vi "ZE_Recorder_AddHeaderToFile.vi"(4 "property values":string[](array[string]), 6 "property names":string[](array[string]), 7 "Header in":string, 8 "error in":errorcluster caption="error in (no error)", 9 "File Type":enum32{"CSV", "TDMS"}(ring), 10 "tdms refnum":refnum<k34>, 11 "csv refnum in":refnum<file>) -> (0 "error out":errorcluster)   [LabVIEW 2025, in "ZE_Recorder.lvlib"]
doc: "ZE_Recorder_AddHeaderToFile.vi\n----------------------------------------------\nThe VI adds a file header containing the measurement information to a CSV or TDMS file.\n\nInputs:\n---------------------\n- property values : 1DArrayOfString; \n- property names : 1DArrayOfString; \n- Header in : String; \n- error in (no error) : Cluster; \n- File Type : EnumU32; \n- tdms refnum : Refnum; \n- csv refnum in : Refnum; \n\nOutputs:\n---------------------\n- error out : Cluster; \n\n----------------------------------------------\n13.06.2016\nZühlke Engineering AG\nCH-8952 Schlieren\nwww.zuehlke.com"
uses:
  ZE_Recorder.lvlib
panel:
  # "Connector Pane"
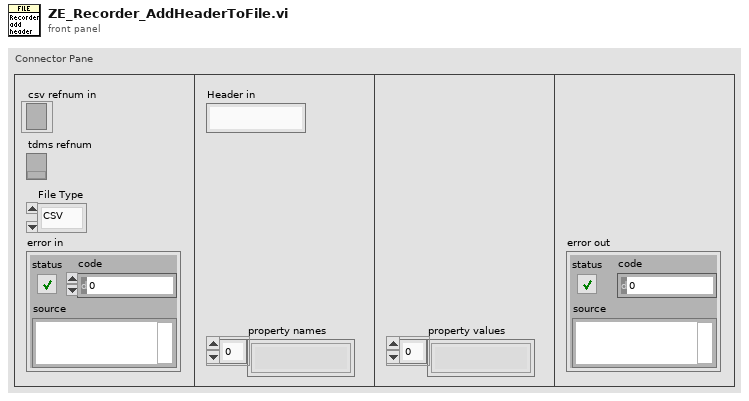
[diagram p1: front panel]
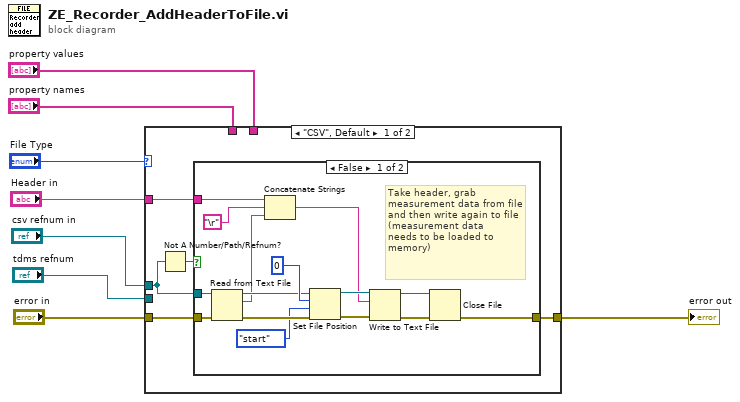
[diagram p0: block diagram]
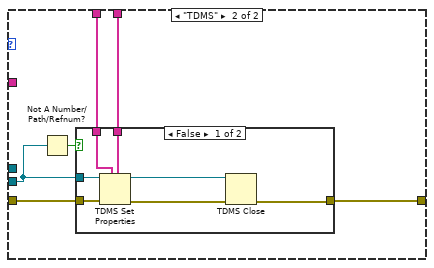
[diagram p3: hidden frame]
diagram:
  n1 = case shown="\"CSV\", Default" "File Type" {
    tunnel: "csv refnum in" -> [w10 _]
    tunnel: "error in" -> [w12 w34]
    tunnel: [w13 w35] -> w6
    tunnel: "tdms refnum" -> [_ w31]
    tunnel: "Header in" -> [w11 _]
    tunnel: "property values" -> [_ w33]
    tunnel: "property names" -> [_ w32]
    frame "CSV", Default {
      n2 = Not A Number/Path/Refnum?(number/path/refnum=w10) -> (NaN/Path/Refnum?=w9:bool)
      n3 = case shown="False" w9 {
        tunnel: [w28 w29] -> w13
        tunnel: w12 -> [w22 w29]
        tunnel: w11 -> [w18 _]
        tunnel: w10 -> [w14 _]
        frame False {
          # "Take header, grab measurement data from file and then write again to file (measurement data \nneeds to be loaded to memory)"
          n4 = Read from Text File(file (use dialog)=w14, error in=w22) -> (refnum out=w21:refnum<file>, text=w19:string, error out=w20:errorcluster)  [unwired: 2 in, 1 out]
          n5 = Concatenate Strings(w18, "\r", w19) -> (w16:string)
          n6 = Set File Position(offset (in bytes) (0)=i64 0, refnum=w21, from (0:start)=enum16{"start", "end", "current"}."start", error in=w20) -> (refnum out=w26:refnum<file>, error out=w25:errorcluster)
          n7 = Write to Text File(file (use dialog)=w26, text=w16, error in=w25) -> (refnum out=w24:refnum<file>, error out=w23:errorcluster)  [unwired: 1 in, 1 out]
          n8 = Close File(refnum=w24, error in=w23) -> (error out=w28:errorcluster)  [unwired: 1 out]
        }
        frame True {
        }
      }
    }
    frame "TDMS" {
      n9 = Not A Number/Path/Refnum?(number/path/refnum=w31) -> (NaN/Path/Refnum?=w30:bool)
      n10 = case shown="False" w30 {
        tunnel: [w42 w43] -> w35
        tunnel: w34 -> [w41 w43]
        tunnel: w33 -> [w40 _]
        tunnel: w32 -> [w39 _]
        tunnel: w31 -> [w36 _]
        frame False {
          n11 = TDMS Set Properties(5:w40, 7:w39, 8:w41, 11:w36) -> (0:w37:errorcluster, 3:w38:refnum<k34>)  [unwired: 2 in, 2 out]
          n12 = TDMS Close(8:w37, 11:w38) -> (0:w42:errorcluster)  [unwired: 1 out]
        }
        frame True {
        }
      }
    }
  }
  "error out" <- w6
